vi "Configure Timebase Reference.vi"(8 "error in (no error)":errorcluster, 9 "Vernier  (F: Disable)":bool, 10 "Reference (1: Center)":u16(ring)=1 items=["Left", "Center", "Right"], 11 "VISA resource name":refnum<visa-resource-name>) -> (0 "error out":errorcluster, 3 "VISA resource name out":refnum<visa-resource-name>)   [LabVIEW 2017, in "Agilent 6000 Series.lvlib"]
doc: "This VI configures reference and vernier."
uses:
  <instrlib>/Agilent 6000 Series/Agilent 6000 Series.lvlib
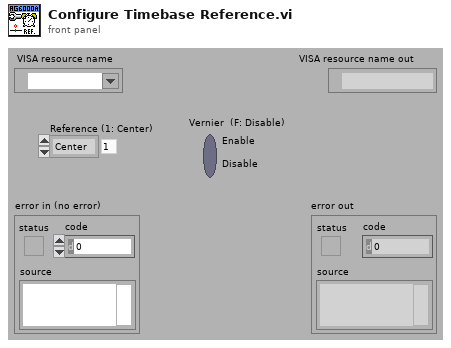
[diagram p1: front panel]
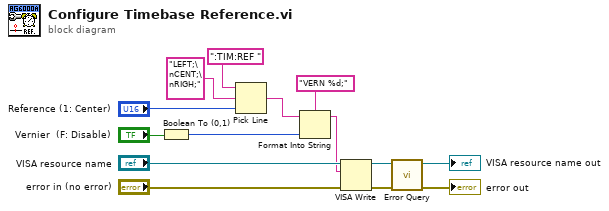
[diagram p0: block diagram]
diagram:
  n1 = Boolean To (0,1)(Boolean="Vernier  (F: Disable)") -> (0, 1=w2:i16)
  n2 = Pick Line(string ("")=":TIM:REF ", multi-line string="LEFT;\nCENT;\nRIGH;", line index="Reference (1: Center)") -> (output string=w4:string)
  n3 = Format Into String(format string="VERN %d;", initial string=w4, w2) -> (resulting string=w1:string)  [unwired: 1 in, 1 out]
  n4 = VISA Write(VISA resource name="VISA resource name", write buffer=w1, error in (no error)="error in (no error)") -> (VISA resource name out=w10:refnum<visa-resource-name>, error out=w9:errorcluster)  [unwired: 1 out]
  n5 = call <instrlib>:"Error Query.vi"("error in (no error)"=w9, "VISA resource name"=w10) -> ("error out"=→"error out":errorcluster, "VISA resource name out"=→"VISA resource name out":refnum<visa-resource-name>)  [unwired: 6 in, 2 out]
